vi "IMAQ-Dispose.vi"(0 "Image Device IN":cluster{"Image":T1, "errorImage":errorcluster}) -> ()   [LabVIEW 2010]
uses:
  <vilib>/vision/Image Controls.llb/IMAQ Image.ctl
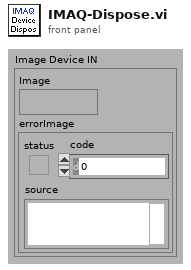
[diagram p1: front panel]
types:
  T1 = typedef "IMAQ Image.ctl" = refnum<image>
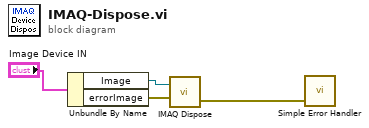
[diagram p0: block diagram]
diagram:
  n1 = Unbundle By Name("Image Device IN") -> ("Image"=w2:T1, "errorImage"=w1:errorcluster)
  n2 = call "IMAQ Dispose"("Image"=w2, "error in (no error)"=w1) -> ("error out"=w3:errorcluster)  [unwired: 4 in]
  n3 = call <vilib>:"Simple Error Handler.vi"("error in (no error)"=w3) -> ()  [unwired: 4 in, 5 out]
